vi "myRIO_BRig_RT_dataAnalog_init.vi"() -> (3 "output_dataAnalog":u16[][](array[numeric]))   [LabVIEW 2014]
panel:
  # "0 - iBlock\n1 - iTrial\n2 - iEvent\n3 - iState at read\n4 - Value AI0\n5 - Value AI1"
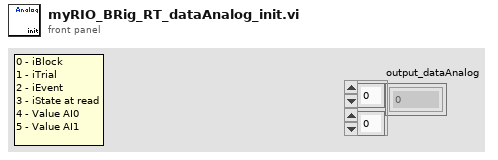
[diagram p1: front panel]
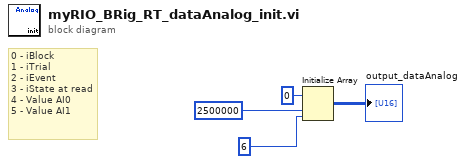
[diagram p0: block diagram]
diagram:
  # "0 - iBlock\n1 - iTrial\n2 - iEvent\n3 - iState at read\n4 - Value AI0\n5 - Value AI1"
  n1 = Initialize Array(u16 0 ("element"), 2500000 ("dimension size"), 6 ("dimension size")) -> (→"output_dataAnalog":u16[][])
